vi "SyncWriteCommand.vi"(7 "MxID":u8=1 format="%x", 8 "error in":errorcluster, 11 "PosParm":i16[](array[numeric])=[0, 0, 0, 0, 0, 0]) -> (0 "error out":errorcluster, 3 "Data":u8[](array[numeric]))   [LabVIEW 2015]
panel:
  out "Sum":u8
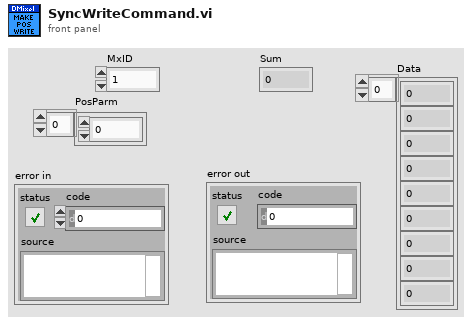
[diagram p1: front panel]
types:
  T1 = cluster{"MxID":u8, u8, u8, u8, u8, u8, u8, u8, u8, u8, u8, u8, u8, u8, u8, u8, u8, u8}
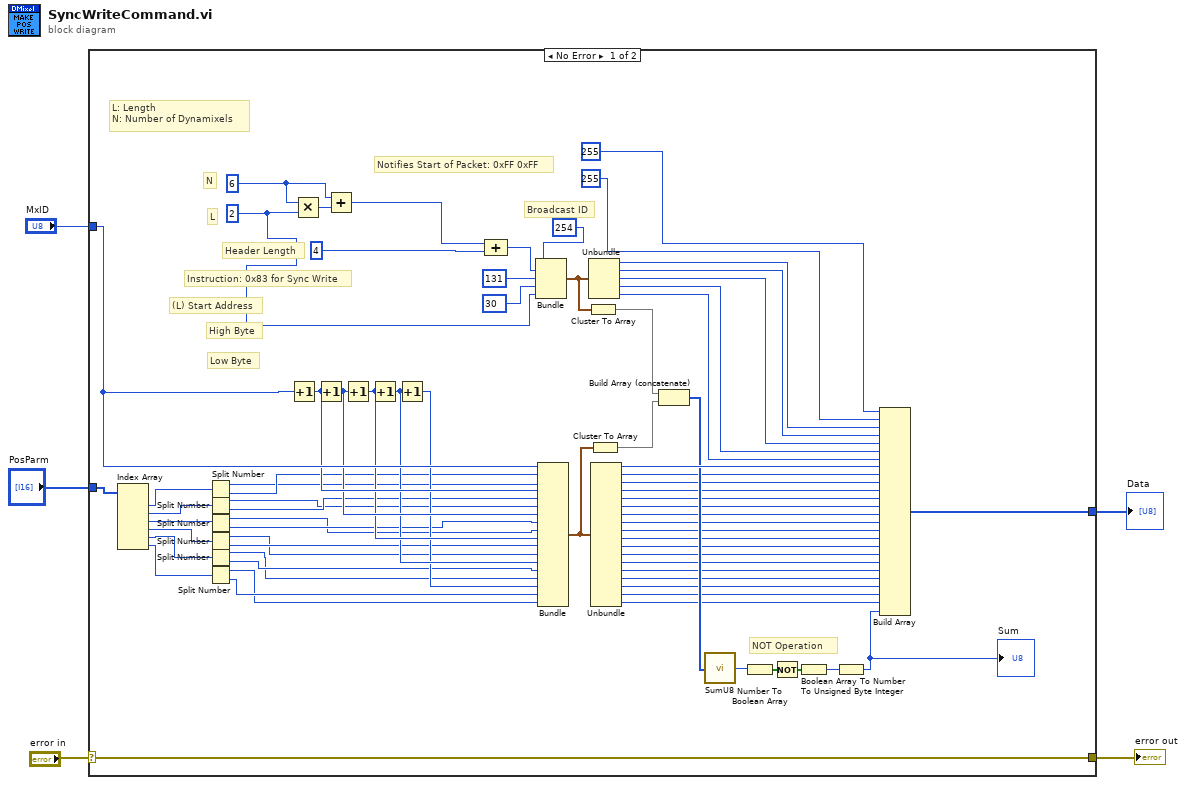
[diagram p0: block diagram]
diagram:
  n1 = case shown="No Error" "error in" {
    selector: "error in" -> [w60 w77]
    tunnel: [w66 _] -> w3
    tunnel: "MxID" -> [w48 _]
    tunnel: [w60 w77] -> w2
    tunnel: "PosParm" -> [w59 _]
    frame No Error {
      w49 = u8 2 ("y")
      w52 = u8 6 ("N")
      # "Instruction: 0x83 for Sync Write"
      # "NOT Operation"
      # "L"
      # "Low Byte"
      # "High Byte"
      # "L: Length \nN: Number of Dynamixels"
      # "Header Length"
      # "N"
      # "(L) Start Address"
      # "Broadcast ID"
      # "Notifies Start of Packet: 0xFF 0xFF"
      n2 = Index Array(array=w59) -> (element #1=w58:i16, element #2=w57:i16, element #3=w56:i16, element #4=w55:i16, element #5=w54:i16, element #6=w53:i16)  [unwired: 6 in]
      n3 = Split Number(x=w58) -> (hi(x)=w16:u8, lo(x)=w17:u8)
      n4 = Split Number(x=w57) -> (hi(x)=w14:u8, lo(x)=w15:u8)
      n5 = Split Number(x=w56) -> (hi(x)=w12:u8, lo(x)=w13:u8)
      n6 = Split Number(x=w55) -> (hi(x)=w10:u8, lo(x)=w11:u8)
      n7 = Split Number(x=w54) -> (hi(x)=w8:u8, lo(x)=w9:u8)
      n8 = Split Number(x=w53) -> (hi(x)=w6:u8, lo(x)=w7:u8)
      n9 = Increment(x=w48) -> (x+1=w22:u8)
      n10 = Multiply(x=w52, y=w49) -> (x*y=w51:u8)
      n11 = Increment(x=w22) -> (x+1=w21:u8)
      n12 = Add(x=w52, y=w51) -> (x+y=w50:u8)
      n13 = Increment(x=w21) -> (x+1=w20:u8)
      n14 = Increment(x=w20) -> (x+1=w19:u8)
      n15 = Increment(x=w19) -> (x+1=w18:u8)
      n16 = Compound Arithmetic op=unknown(w50, u8 4 ("value")) -> (w76:u8)
      n17 = Bundle("MxID"=u8 254, w76, u8 131, u8 30, "y"=w49) -> (w65:cluster{"MxID":u8, u8, u8, u8, "y":u8})  [unwired: 1 in]
      n18 = Bundle("MxID"=w48, w17, w16, w22, w15, w14, w21, w13, w12, w20, w11, w10, w19, w9, w8, w18, w7, w6) -> (w47:T1)  [unwired: 1 in]
      n19 = Cluster To Array(cluster=w65) -> (array=w46:u8[])
      n20 = Unbundle(w65) -> ("MxID"=w67:u8, w68:u8, w69:u8, w70:u8, "y"=w42:u8)
      n21 = Cluster To Array(cluster=w47) -> (array=w45:u8[])
      n22 = Unbundle(w47) -> ("MxID"=w71:u8, w41:u8, w40:u8, w39:u8, w38:u8, w37:u8, w36:u8, w35:u8, w34:u8, w33:u8, w32:u8, w31:u8, w30:u8, w29:u8, w28:u8, w27:u8, w26:u8, w25:u8)
      n23 = Build Array (concatenate)(w46, w45) -> (w44:u8[])
      n24 = call "SumU8.vi"("Array"=w44) -> ("Sum"=w43:u8)
      n25 = Number To Boolean Array(number=w43) -> (Boolean array=w64:bool[])
      n26 = Not(x=w64) -> (.not. x?=w63:bool[])
      n27 = Boolean Array To Number(Boolean array=w63) -> (number=w24:u8)
      n28 = To Unsigned Byte Integer(number=w24) -> (unsigned 8bit integer=w23:u8)
      "Sum" <- w23
      n29 = Build Array(u8 255, u8 255, w67, w68, w69, w70, w42, w71, w41, w40, w39, w38, w37, w36, w35, w34, w33, w32, w31, w30, w29, w28, w27, w26, w25, w23) -> (w66:u8[])
    }
    frame Error {
    }
  }
  "error out" <- w2
  "Data" <- w3
